vi "Log gRPC Data.vi"(8 "error in (no error)":errorcluster, 9 "Value":string, 10 "LogMessageFrequency":T2, 11 "LogMessageSize":T1) -> (0 "error out":errorcluster)   [LabVIEW 2019, in "gRPC Template Creation Utility.lvlib"]
uses:
  gRPC Template Creation Utility.lvlib
  <vilib>/UDC/niceiplib.lvlib
  <vilib>/UDC/Controls/LogMessageFrequency.ctl
  <vilib>/UDC/Controls/LogMessageSize.ctl
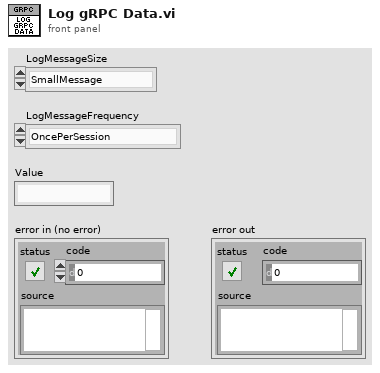
[diagram p1: front panel]
types:
  T1 = typedef "niceiplib.lvlib/LogMessageSize.ctl" = enum32{"SmallMessage", "MediumMessage", "LargeMessage"}
  T2 = typedef "niceiplib.lvlib/LogMessageFrequency.ctl" = enum32{"OncePerSession", "LowFrequency", "MediumFrequency", "HighFrequency", "KBMouseEvents"}
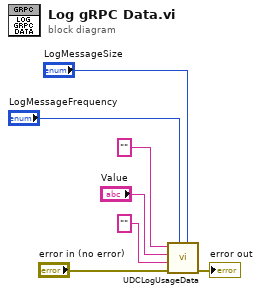
[diagram p0: block diagram]
diagram:
  n1 = call <vilib>:"UDCLogUsageData.vi"("LogMessageSize"="LogMessageSize", "LogMessageFrequency"="LogMessageFrequency", "Error In"="error in (no error)", "KeyUID"="", "Value"="Value", "Key"="") -> ("Error Out"=→"error out":errorcluster)  [unwired: 5 in]
